vi "PicoScope3000aExampleStreamingMSO.vi"() -> ()   [LabVIEW 2010]
doc: "This example demonstrates how to use the PicoScope Labview library to stream data from a PicoScope 5000 Series Device"
uses:
  <vilib>/Waveform/DWDTOps.llb/DWDT Analog to Digital.vi
  ps3000aWrap.dll
  PicoScope3000aLib/PicoScope3000aAnalogChannelSettings.ctl
  PicoScope3000aLib/PicoScope3000aDigitalChannelSettings.ctl
  shared/Buffer and Transfer Settings.ctl
panel:
  out "Device Info":T1
  in  "Write ChA to file":bool
  in  "Port 0 Settings":T2={"Enabled"=FALSE, "Logic Level"=9830} {"Logic Level" items=["1.5V TTL"=9830, "2.5V CMOS"=16383]}
  in  "Trigger Settings":T3={"Trigger Enabled"=FALSE, "Trigger Source"=enum."Channel A", "Trigger Threshold (volts)"=0.0, "Trigger Direction"=2, "Trigger Delay (samples)"=0, "Auto Trigger Time (ms)"=1000} {"Trigger Direction" items=["Above", "Below", "Rising", "Falling", "Rising or Falling"]}
  in  "Channel A Settings":T4={"Enabled"=TRUE, "Coupling"=1, "Range"=6, "Analogue Offset"=0.0, "Bandwidth Limit"=0} {"Bandwidth Limit" items=["Full", "20MHz"]; "Range" items=["10 mV", "20 mV", "50 mV", "100 mV", "200 mV", "500 mV", "1 V", "2 V", "5 V", "10 V", "20 V", "50 V ", "100 V"]; "Coupling" items=["AC", "DC"]}
  out "Analog Channels":T5(graph)
  out "Raw Sample Interval (sec)":dbl=1.0000000130088963e-06 format="%#.5p"
  out "Max ADC value":i16
  out "Chunk time":u32
  out "Elapsed time":dbl
  in  "Data file":path=path "PicoScope3000aExampleStreaming ChA Data"
  out "size(s)":i32
  out "Queue depth":i32(graph)
  out "queue depth":i32
  in  "Buffer and Transfer Settings":T6={"startIndex"=0, "Samples"=1000000, "Down Sample Ratio"=1, "Down-Sample Mode"=0} {"Down-Sample Mode" items=["RAW none"=2147483648, "None"=0, "Aggregate"=1, "Decimate"=2, "Average"=4]; "Down Sample Ratio" step=1; "Samples" format="%_6p"}
  out "USB Powered":bool=TRUE
  out "USB 3.0 device on non-USB 3.0 Port":bool=TRUE
  out "TriggeredAt (In Buffer)":u32 format="%#.6p"
  out "TriggeredAt (Total samples)":u32 format="%#.6p"
  in  "Acquisition Settings":T7={"Auto Stop"=TRUE, "Desired Sample Interval"=1, "Pre-trigger Samples"=0, "Post-trigger Samples"=1000000, "Down-Sample Ratio"=1, "Down-Sample Mode"=0, "Time Units"=3} {"Time Units" items=["Nanoseconds (ns)"=2, "Microseconds (us)"=3, "Milliseconds (ms)"=4, "Seconds (s)"=5]; "Down-Sample Mode" items=["None"=0, "Aggregate"=1, "Decimate"=2, "Average"=4]; "Post-trigger Samples" format="%#.6p"; "Pre-trigger Samples" format="%#_6p"}
  out "Port 0":digitalwaveform(graph)={"t0"=timestamp(0 s since 1904-01-01), "dt"=1.0000000130088963e-06, "Y"={"transitions"=[], "data"=[]}}
  out "Triggered":bool
  out "DownSample Interval (sec)":dbl=1.0000000130088963e-06 format="%#.5p"
  out "Total Samples":u32 format="%#.6p"
  out "Auto Stopped":bool
  in  "Serial Number":string
  in  "Open Using Serial Number":bool
  out "Number of Samples per Capture":u32 format="%#.6p"
  in  "Apply  Settings":bool
  in  "stop":bool
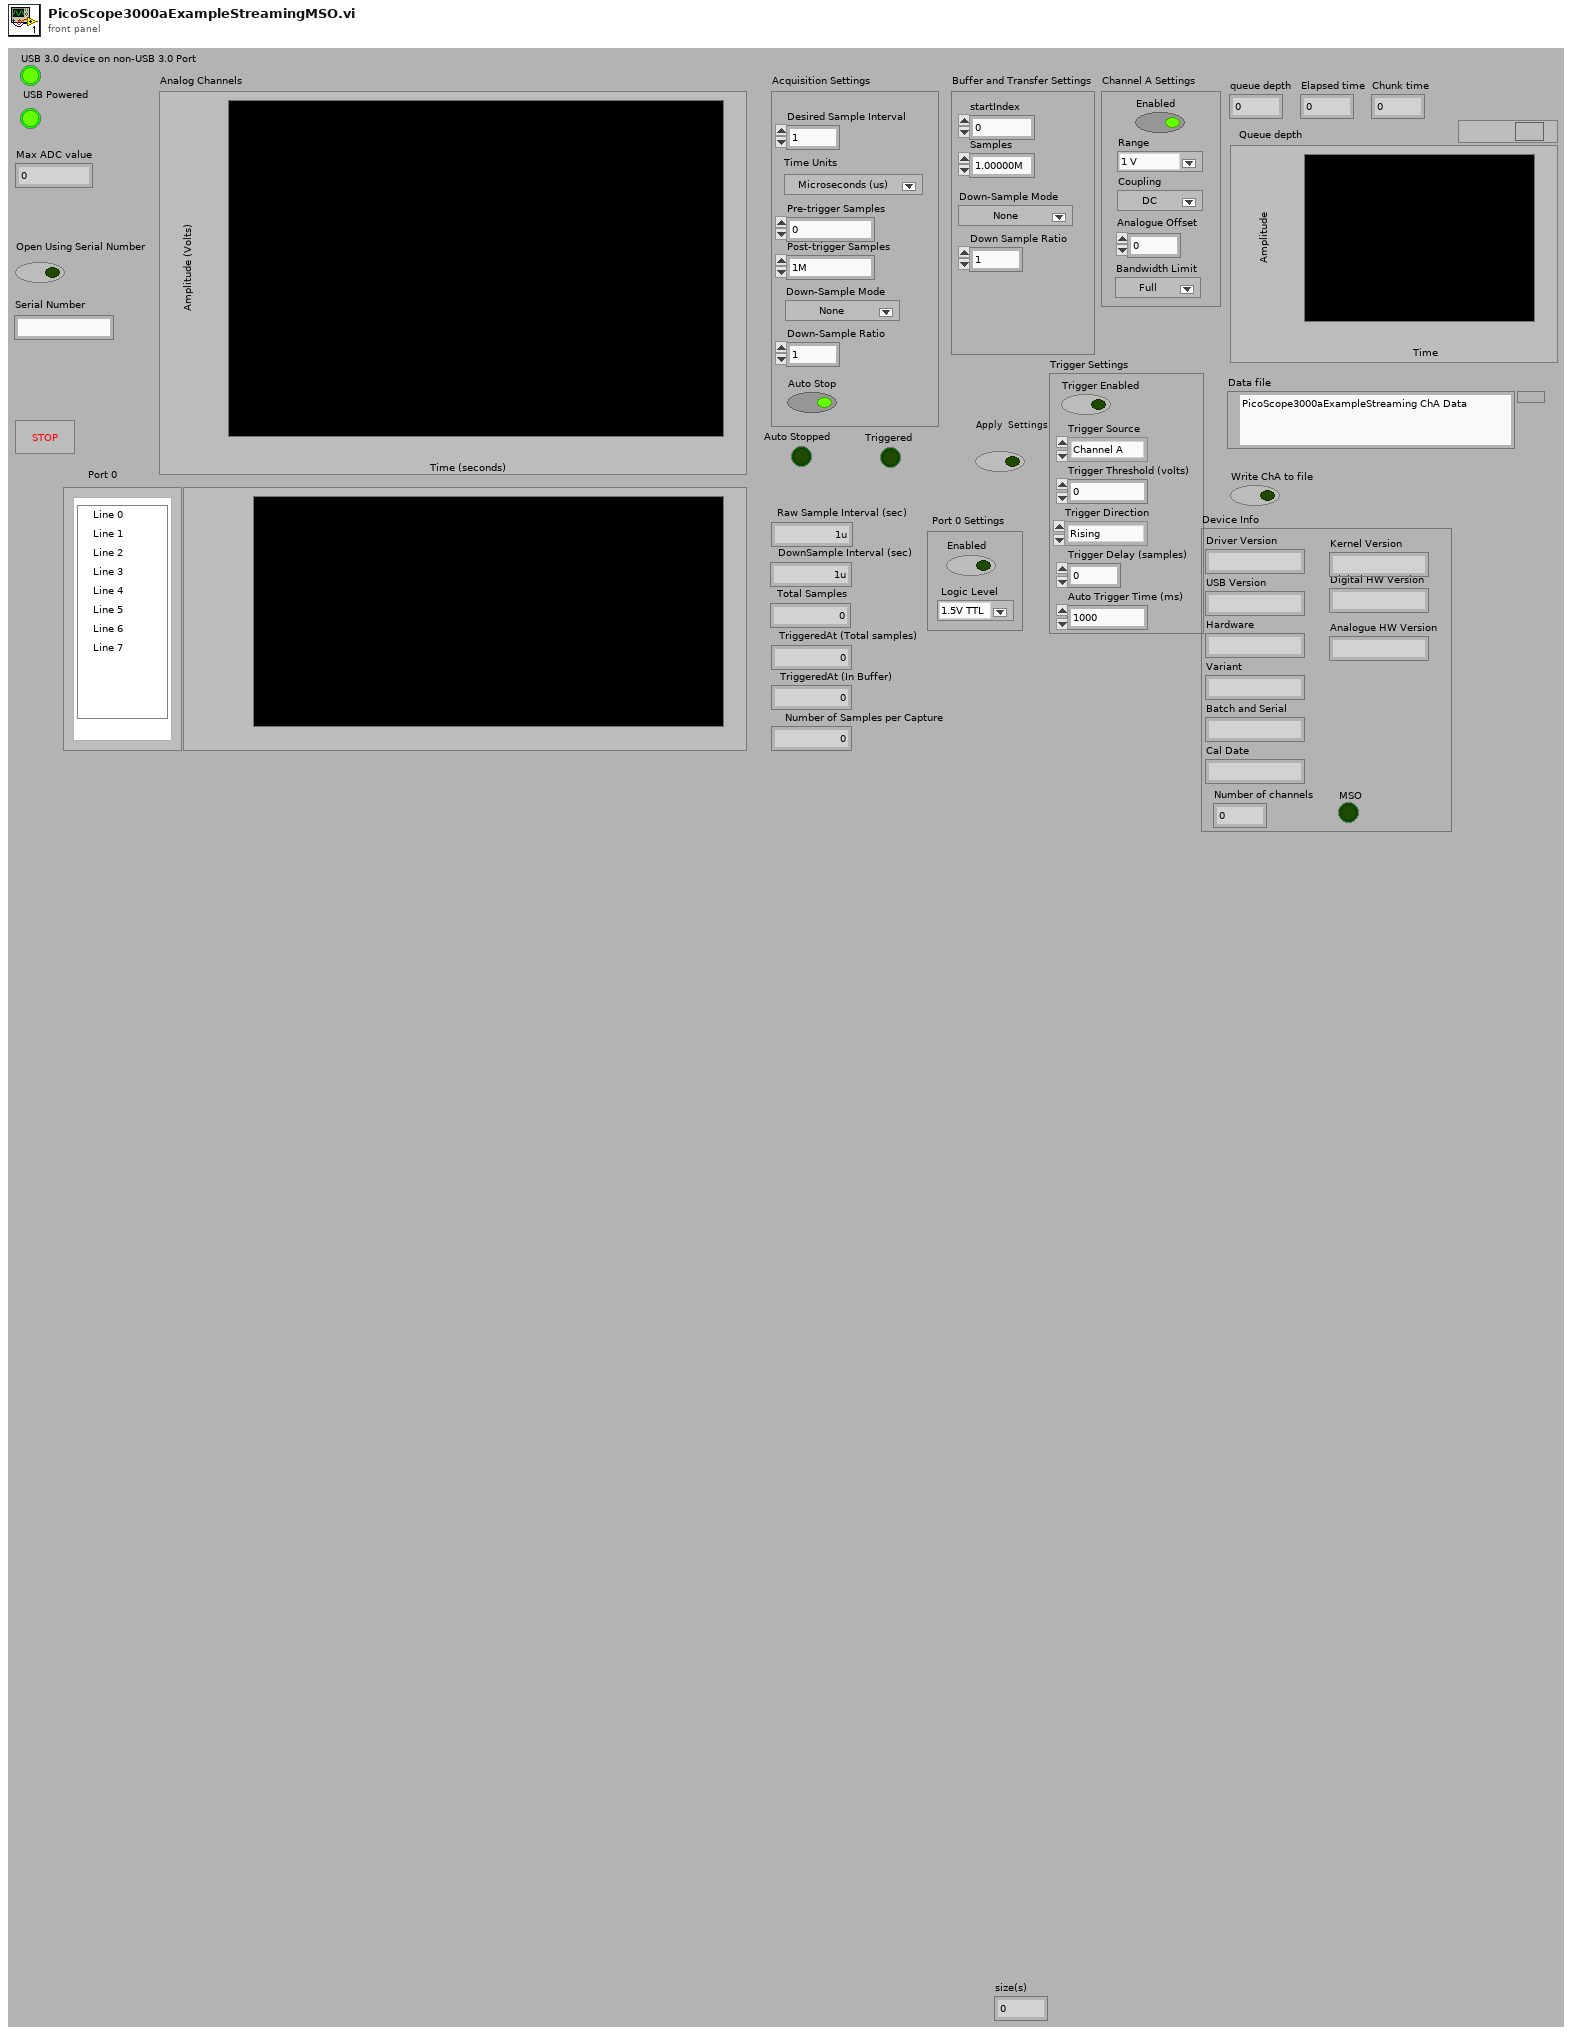
[diagram p1: front panel]
types:
  T1 = cluster{"Driver Version":string, "USB Version":string, "Hardware":string, "Variant":string, "Batch and Serial":string, "Cal Date":string, "Kernel Version":string, "Digital HW Version":string, "Analogue HW Version":string, "MSO":bool, "Number of channels":i16}
  T2 = typedef "PicoScope3000aDigitalChannelSettings.ctl" = cluster{"Enabled":bool, "Logic Level":i16}
  T3 = cluster{"Trigger Enabled":bool, "Trigger Source":enum32{"Channel A", "Channel B", "Channel C", "Channel D", "Ext."}, "Trigger Threshold (volts)":dbl, "Trigger Direction":u32, "Trigger Delay (samples)":u32, "Auto Trigger Time (ms)":i16}
  T4 = typedef "PicoScope3000aAnalogChannelSettings.ctl" = cluster{"Enabled":bool, "Coupling":u32, "Range":u32, "Analogue Offset":sgl, "Bandwidth Limit":u32}
  T5 = cluster{i32, "DownSample Interval (sec)":dbl, "Data":dbl[]}
  T6 = typedef "Buffer and Transfer Settings.ctl" = cluster{"startIndex":u64, "Samples":u64, "Down Sample Ratio":u64, "Down-Sample Mode":u32}
  T7 = cluster{"Auto Stop":bool, "Desired Sample Interval":u32, "Pre-trigger Samples":u32, "Post-trigger Samples":u32, "Down-Sample Ratio":u32, "Down-Sample Mode":i32, "Time Units":u32}
  T8 = enum16{"open", "open or create", "create or replace", "create", "open (read-only)"}
  T9 = cluster{"Channel A Buffer":i16[], "Channel B Buffer":i16[], "Channel C Buffer":i16[], "Channel D Buffer":i16[], "Channel E Buffer":i16[], "Channel F Buffer":i16[], "Channel G Buffer":i16[], "Channel H Buffer":i16[], "Port 0":i16[], "Port 1":i16[]}
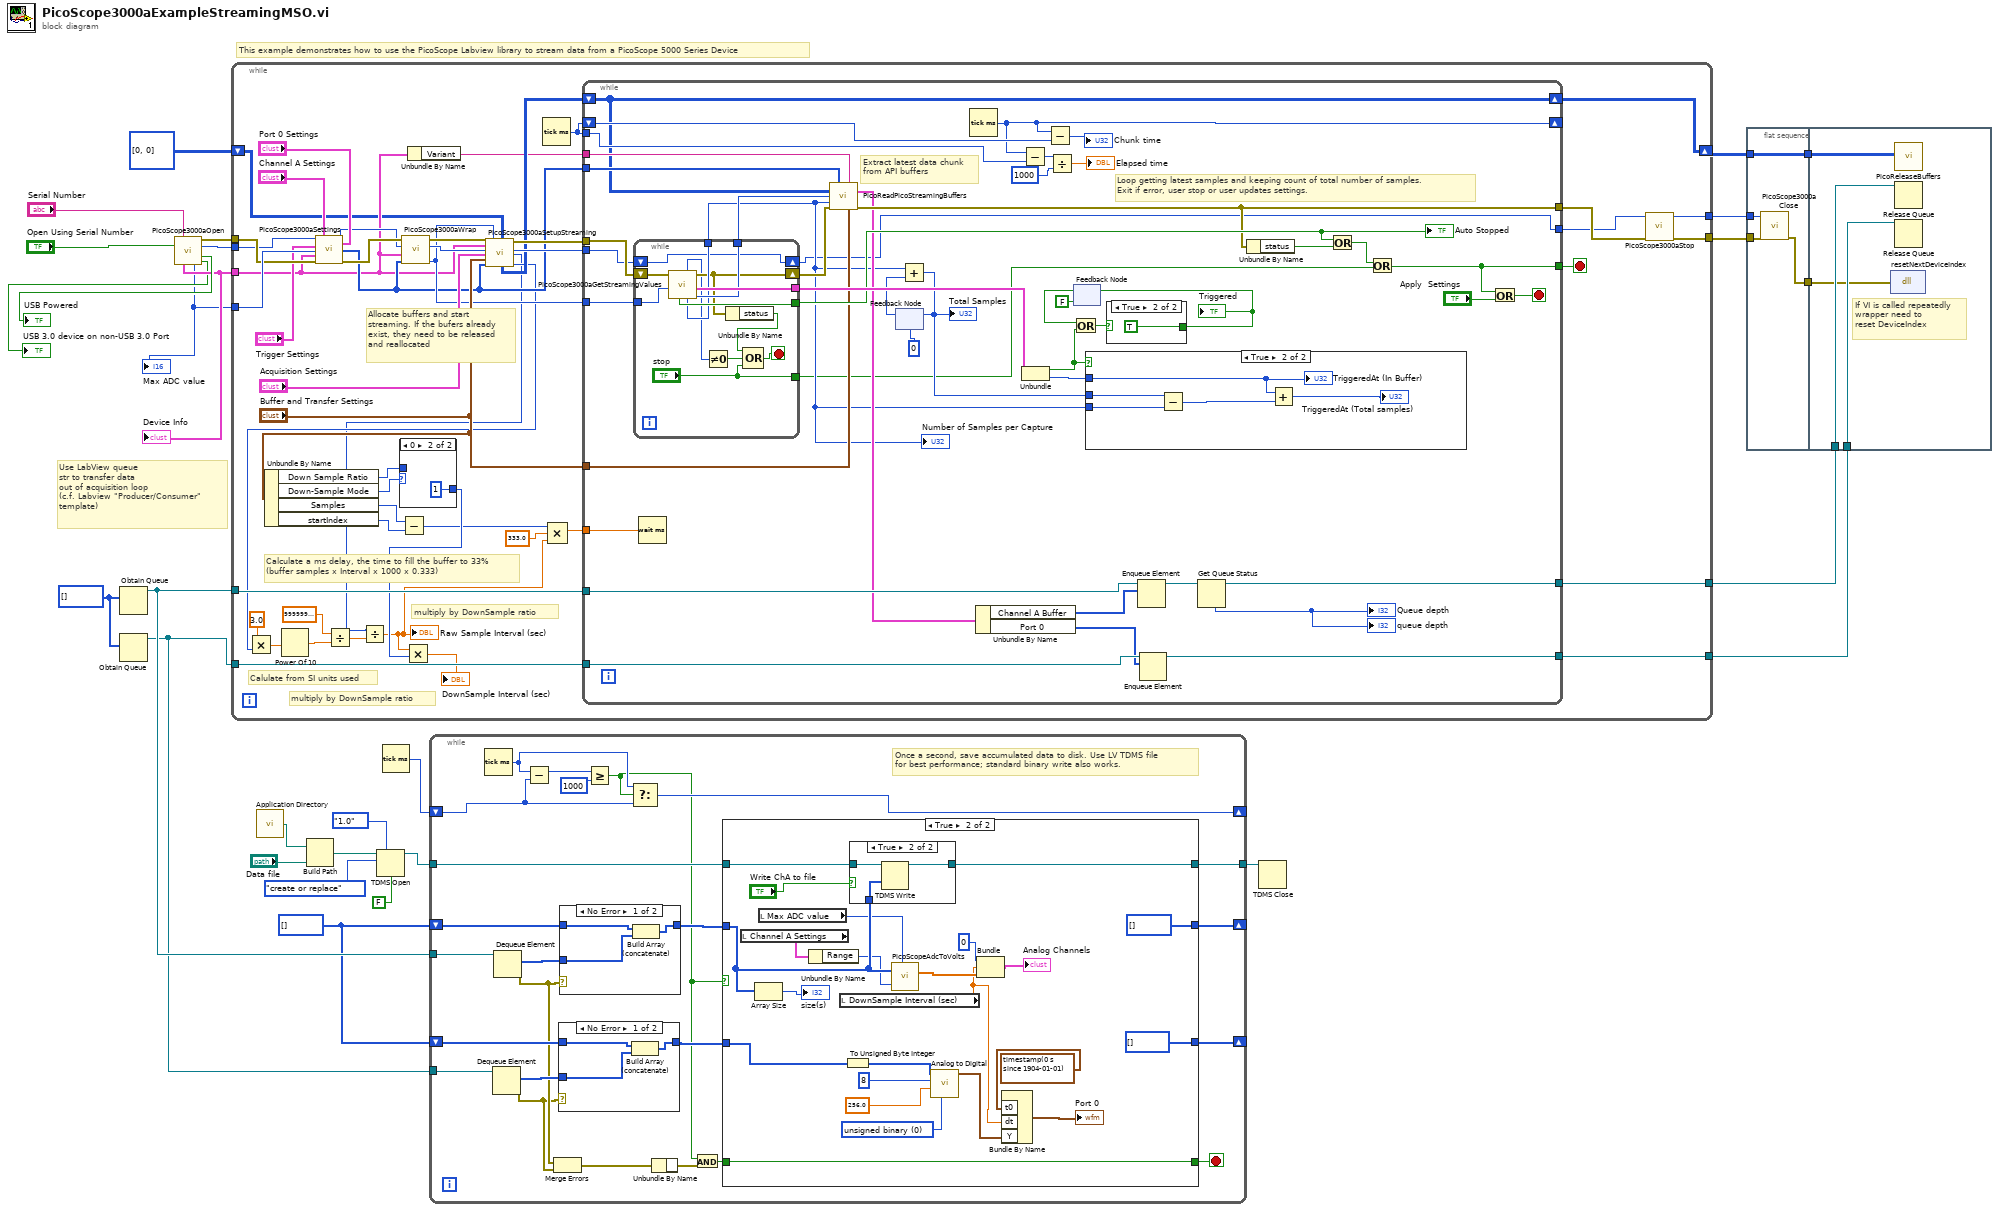
[diagram p0: block diagram]
diagram:
  w12 = i16[] [] ("History Data")
  w15 = i16[] [] ("History Data")
  # "Use LabView queue\nstr to transfer data\nout of acquisition loop\n(c.f. Labview \"Producer/Consumer\"\ntemplate)"
  # "This example demonstrates how to use the PicoScope Labview library to stream data from a PicoScope 5000 Series Device"
  n1 = Obtain Queue(element data type=w15) -> (queue out=w25:refnum<queue>)  [unwired: 4 in, 2 out]
  n2 = Obtain Queue(element data type=w15) -> (queue out=w13:refnum<queue>)  [unwired: 4 in, 2 out]
  n3 = call "PicoScope3000aOpen.vi"("Serial Number"="Serial Number", "Use Serial number"="Open Using Serial Number") -> ("error out"=w29:errorcluster, "handle"=w28:i16, "USB Powered"=→"USB Powered":bool, "Device Info"=w8:T1, "Max ADC value"=w6:i16, "USB 3.0 device on non-USB 3.0 Port"=→"USB 3.0 device on non-USB 3.0 Port":bool)  [unwired: 7 in, 1 out]
  "Max ADC value" <- w6
  "Device Info" <- w8
  n4 = while {
    tunnel: [w33] -> w24
    tunnel: w29 -> [w59]
    tunnel: w28 -> [w58]
    tunnel: w8 -> [w36]
    tunnel: w6 -> [w63]
    tunnel: [w69] -> w23
    tunnel: w25 -> [w68]
    tunnel: [w66] -> w14
    tunnel: w13 -> [w65]
    tunnel: [w32] -> w5
    shift-right: [w30] -> w2
    shift-left: u64[][] [[0], [0]] ("Pointer array") -> [w31]
    stop <- w77 stop-if-true
    # "multiply by DownSample ratio"
    # "Calculate a ms delay, the time to fill the buffer to 33%\n(buffer samples x Interval x 1000 x 0.333)"
    # "Calulate from SI units used"
    # "multiply by DownSample ratio"
    # "Allocate buffers and start\nstreaming. If the bufers already\nexist, they need to be released\nand reallocated"
    n5 = Unbundle By Name("Buffer and Transfer Settings") -> ("Down Sample Ratio"=w72:u64, "Down-Sample Mode"=w73:u32, "Samples"=w45:u64, "startIndex"=w44:u64)
    n6 = call "PicoScope3000aSettings.vi"("handle in"=w58, "Channel A Settings"="Channel A Settings", "Port 0 Settings"="Port 0 Settings", "Trigger Settings"="Trigger Settings", "Max_adc"=w63, "Device Info"=w36, "error in"=w59) -> ("handle out"=w55:i16, "Enabled Array"=w54:i16[], "error out"=w56:errorcluster)  [unwired: 6 in]
    n7 = case shown="0" w73 {
      tunnel: [w78 u32 1 ("Down-Sample Ratio")] -> w43
      tunnel: w72 -> [w78 _]
      frame Default {
      }
      frame 0 {
      }
    }
    n8 = Subtract(x=w45, y=w44) -> (x-y=w42:u64)
    n9 = call "PicoScope3000aWrap.vi"("Enabled Array"=w54, "Device Info"=w36, "handle in"=w55, "error in (no error)"=w56) -> ("deviceIndex"=w60:u16, "handle out"=w61:i16, "error out"=w74:errorcluster)  [unwired: 1 in]
    n10 = Unbundle By Name(w36) -> ("Variant"=w37:string)
    n11 = call "PicoScope3000aSetupStreaming.vi"("error in"=w74, "Device Info"=w36, "handle in"=w61, "Acquisition Settings"="Acquisition Settings", "Buffer and Transfer Settings"="Buffer and Transfer Settings", "enabled array"=w54, "deviceIndex"=w60, "Pointers In"=w31) -> ("Pointer array"=w67:u64[][], "error out"=w75:errorcluster, "handle out"=w76:i16, "Sample Interval"=w46:u32, "sampleIntervalTimeUnits"=w47:u32)  [unwired: 7 in]
    n12 = Multiply(x=3.0, y=w47) -> (x*y=w52:dbl)
    n13 = Power Of 10(x=w52) -> (10^x=w51:dbl)
    n14 = Divide(x=sgl 1000000000000000.0 ("y"), y=w51) -> (x/y=w50:dbl)
    n15 = Divide(x=w46, y=w50) -> (x/y=w38:dbl)
    "Raw Sample Interval (sec)" <- w38
    n16 = Multiply(x=w38, y=w43) -> (x*y=→"DownSample Interval (sec)":dbl)
    n17 = Tick Count (ms)() -> (millisecond timer value=w53:u32)
    n18 = Compound Arithmetic op=MULTIPLY(w42, 333.0 ("value"), w38) -> (w39:dbl)
    n19 = while {
      tunnel: [w84] -> w34
      tunnel: [w124] -> w77
      tunnel: w76 -> [w85]
      tunnel: w75 -> [w109]
      tunnel: [w106] -> w35
      tunnel: "Buffer and Transfer Settings" -> [w108]
      tunnel: w54 -> [w105]
      tunnel: [w103] -> w69
      tunnel: w68 -> [w101]
      shift-right: [w95] -> _
      shift-left: w53 -> [w96]
      tunnel: w37 -> [w90]
      tunnel: [w80] -> w66
      tunnel: w65 -> [w89]
      tunnel: w60 -> [w86]
      tunnel: w53 -> [w83]
      tunnel: w39 -> [w82]
      shift-right: [w81] -> w30
      shift-left: w67 -> [w81]
      stop <- w123 stop-if-true
      # "Loop getting latest samples and keeping count of total number of samples. \nExit if error, user stop or user updates settings."
      # "Extract latest data chunk\nfrom API buffers"
      n20 = while {
        tunnel: [w138] -> w122
        tunnel: [w137] -> w119
        tunnel: [w135] -> w92
        tunnel: [w134] -> w91
        shift-right: [w127] -> w84
        shift-left: w85 -> [w127]
        shift-right: [w133] -> w107
        shift-left: w109 -> [w136]
        tunnel: ["stop"] -> w87
        tunnel: w86 -> [w126]
        stop <- w129 stop-if-true
        n21 = call "PicoScope3000aGetStreamingValues.vi"("deviceIndex"=w126, "error in"=w136) -> ("Start Index"=w135:u32, "Trigger"=w138:cluster{bool, "triggeredAt (Total samples)":u32}, "error out"=w133:errorcluster, "Number of Samples"=w134:i32, "ready"=w132:i16, "Auto Stopped"=w137:bool)  [unwired: 4 in]
        n22 = Not Equal To 0?(x=w132) -> (x != 0?=w130:bool)
        n23 = Unbundle By Name(w133) -> ("status"=w131:bool)
        n24 = Compound Arithmetic op=OR(w131, w130, "stop") -> (w129:bool)
      }
      "Number of Samples per Capture" <- w91
      "Auto Stopped" <- w119
      n25 = Wait (ms)(milliseconds to wait=w82) -> ()  [unwired: 1 out]
      n26 = call "PicoReadPicoStreamingBuffers.vi"("enabled array"=w105, "Buffer and Transfer Settings"=w108, "Variant"=w90, "Pointer array"=w81, "Offset Index"=w92, "Number of Samples"=w91, "error in (no error)"=w107) -> ("Buffers (Max or non-aggregated)"=w100:T9, "error out"=w106:errorcluster)  [unwired: 6 in, 1 out]
      n27 = feedback #1(u32 0) -> (w115:u32)
      n28 = Add(x=w91, y=w115) -> (x+y=w113:u32)
      "Total Samples" <- w113
      n29 = feedback-in #1(w113) -> ()
      n30 = Tick Count (ms)() -> (millisecond timer value=w95:u32)
      n31 = Unbundle By Name(w100) -> ("Channel A Buffer"=w93:i16[], "Port 0"=w88:i16[])
      n32 = Subtract(x=w95, y=w83) -> (x-y=w99:u32)
      n33 = Unbundle(w122) -> (w111:bool, "triggeredAt (Total samples)"=w110:u32)
      n34 = Subtract(x=w95, y=w96) -> (x-y=→"Chunk time":u32)
      n35 = Divide(x=w99, y=u32 1000) -> (x/y=→"Elapsed time":dbl)
      n36 = feedback #2(FALSE) -> (w117:bool)
      n37 = Or(x=w117, y=w111) -> (x .or. y?=w114:bool)
      n38 = case shown="True" w111 {
        tunnel: w91 -> [_ w139]
        tunnel: w113 -> [_ w143]
        tunnel: w110 -> [_ w141]
        frame False {
        }
        frame True {
          n39 = Subtract(x=w143, y=w139) -> (x-y=w142:u32)
          n40 = Add(x=w141, y=w142) -> (x+y=→"TriggeredAt (Total samples)":u32)
          "TriggeredAt (In Buffer)" <- w141
        }
      }
      n41 = case shown="True" w114 {
        selector: w114 -> [w144 _]
        tunnel: [w144 TRUE] -> w112
        frame False {
        }
        frame True {
        }
      }
      "Triggered" <- w112
      n42 = feedback-in #2(w112) -> ()
      n43 = Enqueue Element(queue=w101, element=w93) -> (queue out=w102:refnum<queue>)  [unwired: 2 in, 2 out]
      n44 = Enqueue Element(queue=w89, element=w88) -> (queue out=w80:refnum<queue>)  [unwired: 2 in, 2 out]
      n45 = Get Queue Status(queue=w102) -> (queue out=w103:refnum<queue>, # elements in queue=→"queue depth" →"Queue depth":i32)  [unwired: 2 in, 6 out]
      n46 = Unbundle By Name(w106) -> ("status"=w121:bool)
      n47 = Or(x=w119, y=w121) -> (x .or. y?=w120:bool)
      n48 = Or(x=w120, y=w87) -> (x .or. y?=w124:bool)
      n49 = Or(x=w124, y="Apply  Settings") -> (x .or. y?=w123:bool)
    }
    n50 = call "PicoScope3000aStop.vi"("error in (no error)"=w35, "handle in"=w34) -> ("error out"=w32:errorcluster, "handle out"=w33:i16)  [unwired: 8 in]
  }
  n51 = call <vilib>:"Application Directory.vi"() -> ("Application Directory"=w9:path)
  n52 = Build Path(base path=w9, name or relative path="Data file") -> (appended path=w10:path)
  n53 = TDMS Open(6:FALSE ("disable buffering? (T)"), 7:enum16{"1.0", "2.0"}."1.0" ("file format version (2.0)"), 10:T8."create or replace" ("operation (0:open)"), 11:w10) -> (3:w19:refnum<k34>)  [unwired: 2 in, 1 out]
  n54 = Tick Count (ms)() -> (millisecond timer value=w21:u32)
  n55 = while {
    tunnel: w25 -> [w168]
    shift-right: [w160] -> _
    shift-left: w12 -> [w167]
    shift-right: [w162] -> _
    shift-left: w21 -> [w163]
    tunnel: w19 -> [w159]
    tunnel: [w158] -> w18
    tunnel: w13 -> [w156]
    shift-right: [w153] -> _
    shift-left: w12 -> [w155]
    stop <- w150 stop-if-true
    # "Once a second, save accumulated data to disk. Use LV TDMS file\nfor best performance; standard binary write also works."
    n56 = Tick Count (ms)() -> (millisecond timer value=w164:u32)
    n57 = Dequeue Element(queue=w156) -> (element=w157:i16[], error out=w151:errorcluster)  [unwired: 2 in, 2 out]
    n58 = Dequeue Element(queue=w168) -> (element=w169:i16[], error out=w152:errorcluster)  [unwired: 2 in, 2 out]
    n59 = Subtract(x=w164, y=w163) -> (x-y=w166:u32)
    n60 = Merge Errors(w152, w151) -> (w148:errorcluster)
    n61 = case shown="No Error" w151 {
      tunnel: w155 -> [w172 w173]
      tunnel: [w171 w173] -> w154
      tunnel: w157 -> [w170 _]
      frame No Error {
        n62 = Build Array (concatenate)(w172, w170) -> (w171:i16[])
      }
      frame Error {
      }
    }
    n63 = case shown="No Error" w152 {
      tunnel: w167 -> [w207 w208]
      tunnel: [w206 w208] -> w161
      tunnel: w169 -> [w205 _]
      frame No Error {
        n64 = Build Array (concatenate)(w207, w205) -> (w206:i16[])
      }
      frame Error {
      }
    }
    n65 = Greater Or Equal?(x=w166, y=u32 1000) -> (x >= y?=w147:bool)
    n66 = Select(t=w164, s=w147, f=w163) -> (s? t:f=w162:u32)
    n67 = And(x=w147) -> (y=w146:errorcluster, x .and. y?=w149:bool)
    n68 = Unbundle By Name(w148, w146) -> ()
    n69 = case shown="True" w147 {
      tunnel: w161 -> [w177 w196]
      tunnel: [w177 i16[] [] ("History Data")] -> w160
      tunnel: w159 -> [w176 w198]
      tunnel: [w176 w197] -> w158
      tunnel: w154 -> [w175 w183]
      tunnel: [w175 i16[] [] ("History Data")] -> w153
      tunnel: w149 -> [w174 w179]
      tunnel: [w174 w179] -> w150
      frame False {
      }
      frame True {
        w189 = u16 0 items=["unsigned binary", "offset binary", "2's complement"] ("data format (offset binary)")
        n70 = local read "Channel A Settings"() -> (w180:T4)
        n71 = Array Size(array=w196) -> (size(s)=→"size(s)":i32)
        n72 = local read "Max ADC value"() -> (w192:i16)
        n73 = Unbundle By Name(w180) -> ("Range"=w195:u32)
        n74 = local read "DownSample Interval (sec)"() -> (w184:dbl)
        n75 = To Unsigned Byte Integer(number=w183) -> (unsigned 8bit integer=w188:u8[])
        n76 = case shown="True" "Write ChA to file" {
          tunnel: w198 -> [w201 w204]
          tunnel: [w201 w203] -> w197
          tunnel: w196 -> [_ w202]
          frame False {
          }
          frame True {
            n77 = TDMS Write(0:w204, 9:w202) -> (4:w203:refnum<k34>)  [unwired: 4 in, 3 out]
          }
        }
        n78 = call "PicoScopeAdcToVolts.vi"("Max_adc"=w192, "Range Index"=w195, "Data"=w196) -> ("Data"=w193:dbl[])
        n79 = call-poly <vilib>:"Analog to Digital.vi"("data format (offset binary)"=w189, "full-scale range (pk-pk)"=256.0, "resolution (16 bit)"=8, "analog waveform"=w188) -> ("digital waveform"=w185:digitalwaveform)  [unwired: 4 in, 3 out]
        n80 = Bundle(0, "DownSample Interval (sec)"=w184, "Data"=w193) -> (→"Analog Channels":T5)  [unwired: 1 in]
        n81 = Bundle By Name("t0"=timestamp(0 s since 1904-01-01), "dt"=w184, "Y"=w185) -> (→"Port 0":digitalwaveform)  [unwired: 1 in]
      }
    }
  }
  n82 = TDMS Close(11:w18) -> ()  [unwired: 1 in, 2 out]
  n83 = flat-sequence {
    tunnel: w24 -> [w212]
    tunnel: w5 -> [w211]
    tunnel: [w210] -> w4
    tunnel: w2 -> [w209]
    tunnel: [w209] -> w1
    tunnel: w23 -> [w216]
    tunnel: w14 -> [w215]
    tunnel: w4 -> [w214]
    tunnel: w1 -> [w213]
    frame #0 {
      n84 = call "PicoScope3000aClose.vi"("error in (no error)"=w211, "handle in"=w212) -> ("error out"=w210:errorcluster)  [unwired: 8 in, 1 out]
    }
    frame #1 {
      # "If VI is called repeatedly\nwrapper need to\nreset DeviceIndex"
      n85 = dll-call lib="ps3000aWrap.dll" fn="resetNextDeviceIndex"(error in=w214) -> ()  [unwired: 3 in, 2 out]
      n86 = call "PicoReleaseBuffers.vi"("Pointer array"=w213) -> ()  [unwired: 9 in, 2 out]
      n87 = Release Queue(queue=w216) -> ()  [unwired: 2 in, 3 out]
      n88 = Release Queue(queue=w215) -> ()  [unwired: 2 in, 3 out]
    }
  }
